vi "DHE_DRV_load_application.vi"(0 "fd":i32, 5 "app":i32, 7 "dest":i16, 11 "error in (no error)":errorcluster) -> (4 "fd out":i32, 8 "return value":i32, 10 "error?":bool, 15 "error out":errorcluster)   [LabVIEW 2016]
doc: "This VI closes the I/O interface with the instrument."
uses:
  c/lib/libarcDHE.so
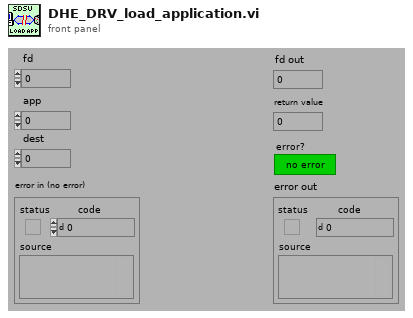
[diagram p1: front panel]
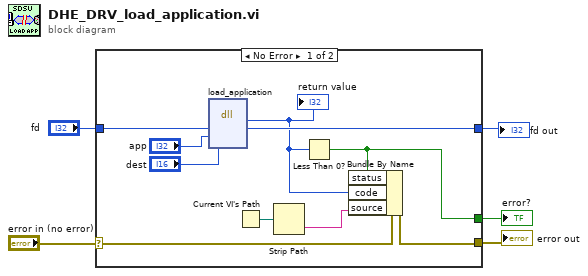
[diagram p0: block diagram]
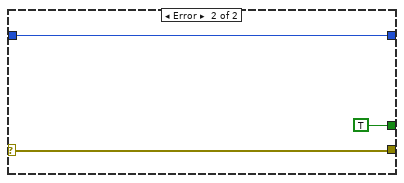
[diagram p2: hidden frame]
diagram:
  n1 = case shown="No Error" "error in (no error)" {
    selector: "error in (no error)" -> [w6 w16]
    tunnel: [w12 w16] -> w5
    tunnel: [w11 TRUE ("error?")] -> w4
    tunnel: "fd" -> [w9 w17]
    tunnel: [w8 w17] -> w2
    frame No Error {
      n2 = dll-call lib="home/simager/panview/PAN/Modules/SDSU/private/c/lib/libarcDHE.so" fn="load_application"("fd"=w9, "app"="app", "dest"="dest") -> (w7:i32, "fd"=w8:i32)  [unwired: 5 in, 2 out]
      "return value" <- w7
      n3 = Current VI's Path() -> (path=w13:path)
      n4 = Strip Path(path=w13) -> (name=w10:string)  [unwired: 1 out]
      n5 = Less Than 0?(x=w7) -> (x < 0?=w11:bool)
      n6 = Bundle By Name(cluster=w6, "status"=w11, "code"=w7, "source"=w10) -> (w12:errorcluster)
    }
    frame Error {
    }
  }
  "error out" <- w5
  "error?" <- w4
  "fd out" <- w2
